vi "02-QNET_MYOELECTRIC_Student_Altered.vi"() -> ()   [LabVIEW 2017]
doc: "This VI is to be used with the QNET Myoelectric Trainer on the NI ELVIS II (or NI ELVIS I)."
uses:
  <vilib>/Simulation/Scripting/Companion Diagram/SimConfigNode/SimDog.xnode
  <vilib>/Simulation/SignalDisplay/Implementation/NILVSim Time Waveform.llb/SIM Time Waveform (vector).vi
  QNET Library/QNET_Drivers.llb/QNET_MYOELECTRIC_Servo_Write.vi
  QNET Library/QNET_Drivers.llb/QNET_MYOELECTRIC_Read_EMG.vi
  <vilib>/Simulation/Implementation/XNodeFramework/SimXNode/SimX.xnode
  <vilib>/Simulation/Implementation/Shared/SIMSCR Execution Mode.ctl
  <vilib>/Simulation/Scripting/Companion Diagram/SimConfigNode/_simSolvers.ctl
  <vilib>/Simulation/Scripting/Companion Diagram/SimConfigNode/SimParams.ctl
  QNET Library/Simulation_Module_Functions/HPF_First_Order_Sim.vi
  QNET Library/Simulation_Module_Functions/LPF_First_Order_Sim.vi
  <vilib>/Simulation/Utility/Implementation/SIM Halt.vi
  <vilib>/Simulation/DiscreteLinear/Implementation/NILVSim Discrete ZOH.llb/SIM Discrete ZOH (scalar).vi
  <vilib>/Simulation/Nonlinear/Implementation/NILVSim DeadZone.llb/SIM DeadZone (scalar).vi
  <vilib>/Simulation/ContinuousLinear/Implementation/NILVSim Integrator new.llb/SIM Integrator (scalar).vi
panel:
  out "output":dbl
  out "x*y":dbl
  in  "Start of Dead Zone":dbl
  in  "Manual Direction":bool
  in  "Servo Command (V)":dbl(knob) min=0.0 max=5.0 step=0.25 scale=0.0..5.0 scale format="%.1f"
  in  "DZ Width (V)":dbl=0.01 min=0.01 max=1.0 step=0.01 format="%_3f"
  in  "Integral Gain":dbl=5.0 min=0.0 max=50.0 step=0.5
  in  "Lower limit (V)":dbl min=0.0 max=10.0 step=0.5
  in  "Upper limit (V)":dbl=5.0 min=0.0 max=10.0 step=0.5
  in  "ZOH Period (s)":dbl=0.5 min=0.01 max=1.0 step=0.01 format="%_3f"
  in  "Threshold (V)":dbl=2.0 min=0.05 max=10.0 step=0.05 format="%_3f"
  in  "LPF Cutoff (Hz)":dbl=25.0 min=0.01 max=200.0 step=0.5 format="%_3f"
  in  "HPF Cutoff (Hz)":dbl=1.0 min=0.01 max=10.0 step=0.05 format="%_3f"
  in  "Tab Control":enum32{"EMG", "Envelope", "Servo"}(tab)
  out "EMG Signals (V)":waveform(dbl)[](graph)=[{"t0"=timestamp(19.448 s since 1904-01-01), "dt"=1.0, "Y"=[5.281750161198542]}, {"t0"=timestamp(19.448 s since 1904-01-01), "dt"=1.0, "Y"=[1.518699315611327e-10]}]
  out "Envelope and ZOH":waveform(dbl)[](graph)=[{"t0"=timestamp(19.448 s since 1904-01-01), "dt"=1.0, "Y"=[1.6271790075730286e-10]}, {"t0"=timestamp(19.448 s since 1904-01-01), "dt"=1.0, "Y"=[1.7286062386519834e-10]}]
  out "Servo Direction and Command":waveform(dbl)[](graph)
  in  "Servo ON/OFF":bool
  out "Direction":bool
  in  "Sampling Rate (Hz)":dbl=100.0 min=0.0 max=1000.0 step=25.0 format="%.1f"
  in  "Device":tag="Dev1"
  in  "Stop":bool
  # "QNET-Myoelectrics"
  # "s"
  # "Servo Control Parameters"
  # "Direction Parameters"
  # "Filtering"
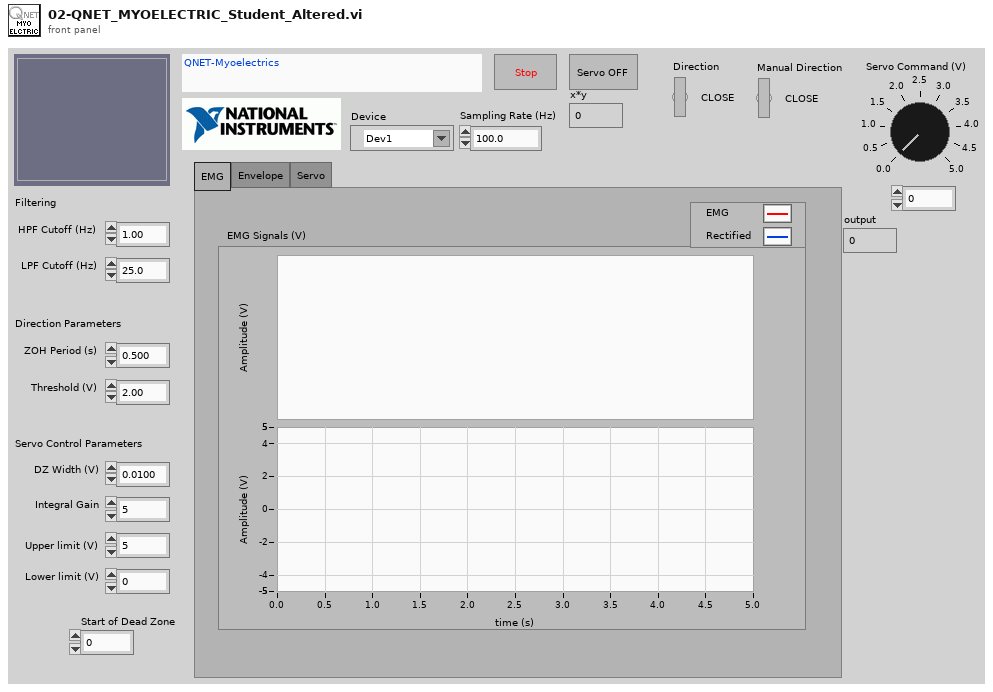
[diagram p1: front panel]
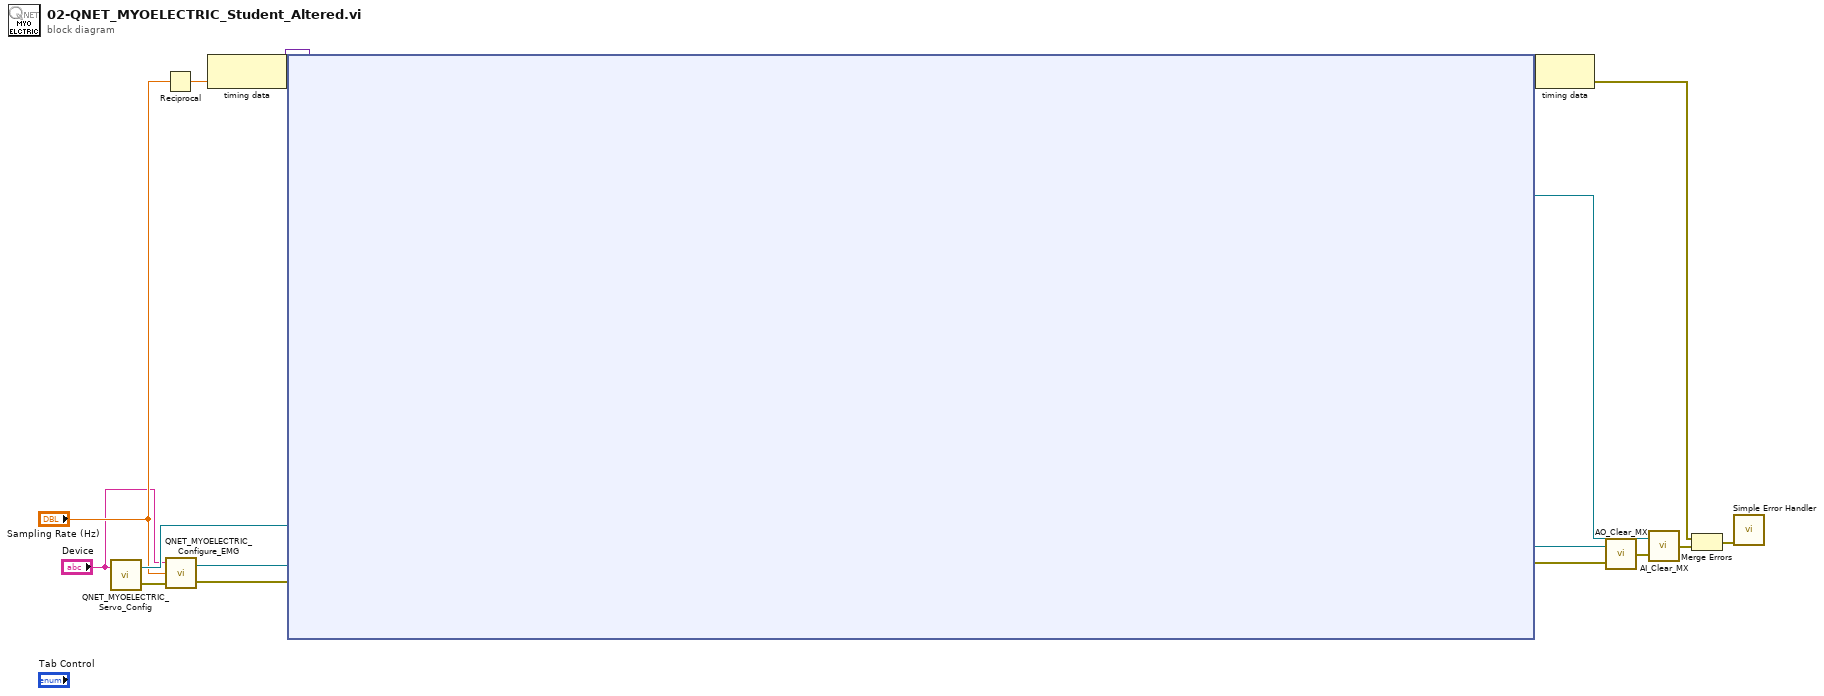
[diagram p0: block diagram]
diagram:
  n1 = call "QNET_MYOELECTRIC_Servo_Config.vi"("dev"="Device") -> ("error out"=w7:errorcluster, "task out"=w14:refnum<k21>)  [unwired: 1 in]
  n2 = Reciprocal(x="Sampling Rate (Hz)") -> (1/x=w6:dbl)
  n3 = call "QNET_MYOELECTRIC_Configure_EMG.vi"("error in"=w7, "Sampling Rate (Hz)"="Sampling Rate (Hz)", "Device"="Device") -> ("error out"=w8:errorcluster, "task out"=w9:refnum<k21>)
  n4 = node-c288(w6) -> (w11:variant)
  n5 = node-c254 ("Simulation Loop")(w11, w14, w9, w8) -> (w10:variant, w16:refnum<k21>, w15:errorcluster, w13:refnum<k21>)
  n6 = node-c288(w10) -> (w4:errorcluster)
  n7 = call "AO_Clear_MX.vi"("Error in"=w15, "Task in"=w16) -> ("Error out"=w12:errorcluster)
  n8 = call "AI_Clear_MX.vi"("Error in"=w12, "Task in"=w13) -> ("Error out"=w3:errorcluster)
  n9 = Merge Errors(w4, w3) -> (w2:errorcluster)
  n10 = call <vilib>:"Simple Error Handler.vi"("error in (no error)"=w2) -> ()  [unwired: 1 in, 8 out]
